vi "test.vi"() -> ()   [LabVIEW 2014]
uses:
  <vilib>/Platform/TimedLoop/XDataNode/timing_clust.ctl
  <vilib>/Platform/TimedLoop/XDataNode/nitl_modes.ctl
  <vilib>/Platform/TimedLoop/XDataNode/wakeup.ctl
  <vilib>/Platform/TimedLoop/XDataNode/XDataNode.xnode
  <vilib>/Platform/TimedLoop/XDataNode/XDNodeRunTimeDep.lvlib
panel:
  out "Signalverlaufsdiagramm":i64(graph)
  out "Globale Endzeit 2":i64
  out "Globale Startzeit":i64
  out "Globale Endzeit":i64
  out "Iterationsdauer":i64
  out "Numerisch":i32
  in  "Stopp":bool
  out "Periode":i64
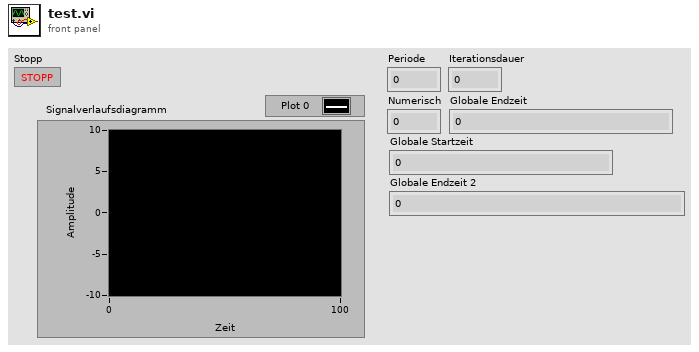
[diagram p1: front panel]
types:
  T1 = typedef "XDNodeRunTimeDep.lvlib/timing_clust.ctl" = cluster{"Expected End [f-1]":u64, "Actual End [f-1]":u64, "Finished Late? [f-1]":bool, "Expected End [i-1]":u64, "Actual End [i-1]":u64, "Finished Late? [i-1]":bool, "Expected Start [i]":u64, "Actual Start [i]":u64, "Expected Start [f]":u64, "Actual Start [f]":u64, "Source Name":string, "Structure Name":string, "Period":i64, "Deadline":i64, "Offset":i64, "Start":i64, "Priority":i32, "Timeout":i32, "Mode":T2, "Wakeup Reason":T3, "Error":errorcluster, "Source Type":string, "Secondary Source Type":string, "Global End Time":u64, "Global Start Time":u64, "Frame Duration":u64, "Iteration Duration":u64, "Assigned CPU":i32, "I/O Scan Engine Mode":u32}
  T2 = typedef "XDNodeRunTimeDep.lvlib/nitl_modes.ctl" = enum32{"No Change", "Process missed periods, maintain original phase", "Discard missed periods, maintain original phase", "Process missed periods, ignore original phase", "Discard missed periods, ignore original phase"}
  T3 = typedef "XDNodeRunTimeDep.lvlib/wakeup.ctl" = enum32{"Normal", "Aborted", "Asynchronous wakeup", "Timing source error", "Timed loop error", "Timeout"}
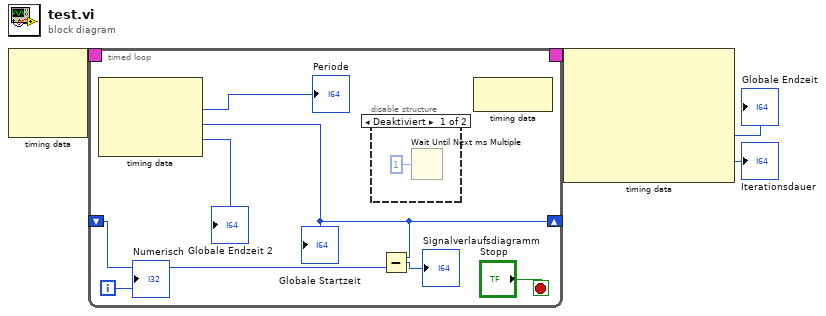
[diagram p0: block diagram]
diagram:
  n1 = node-c288() -> (w4:T1)  [unwired: 4 in]
  n2 = timed-loop {
    timing: w4 -> [_]
    timing-out: [_] -> w3
    shift-right: [w6] -> _
    shift-left: _ -> [w7]
    i -> [w9]
    stop <- "Stopp" stop-if-true
    n3 = node-c288() -> (→"Periode":i64, w6:i64, →"Globale Endzeit 2":i64)  [unwired: 1 in, 1 out]
    "Globale Startzeit" <- w6
    n4 = disable-structure shown="Deaktiviert" {
      frame Disabled {
        n5 = Wait Until Next ms Multiple(millisecond multiple=u32 1 ("ms")) -> ()  [unwired: 1 out]
      }
      frame Enabled {
      }
    }
    n6 = Subtract(x=w6, y=w7) -> (x-y=→"Signalverlaufsdiagramm":i64)
    n7 = node-c288() -> ()  [unwired: 1 in, 1 out]
    "Numerisch" <- w9
  }
  n8 = node-c288(w3) -> (→"Globale Endzeit":i64, →"Iterationsdauer":i64)  [unwired: 5 out]
